vi "niFPGA 3phasePLL.vi"(0 "input (phase value)":T2, 1 "reset":bool, 5 "PI gains":T1={"proportional gain (Kp)"=12.0, "integral gain (Ki)"=200.0}, 7 "anti-windup gain (Ka)":fxp<+,16,9>=200.0, 12 "dt":fxp<+,24,-5>=9.999983012676239e-05) -> (3 "frequency":fxp<+,32,8> format="%.27g", 4 "phase (pi)":fxp<+/-,32,1> format="%.32g", 6 "sin(phase)":fxp<+/-,32,2> format="%.31g", 8 "cos(phase)":fxp<+/-,32,2> format="%.31g")   [LabVIEW 2017]
doc: "Tracks the <B>phase</B> and <B>frequency</B> of a three-phase signal. This operation is useful for FPGA control applications of a three-phase system. The output <B>phase</B> of the 3-Phase Phase-Locked Loop is in pi radians.\n\nTo define the <B>Input mode</B>, double-click this Express VI and use the <B>Input mode</B> control to specify phase value input--<B>input (phase value)</B> or line value input--<B>input (line value)</B>. \n\n\n\nUse this VI in a While Loop."
uses:
  <vilib>/rvi/FXPMathLib/FxpMul/XNode/nifxpmath_Multiplier.xnode
  <vilib>/rvi/FXPMathLib/sim/FxpSim.dll
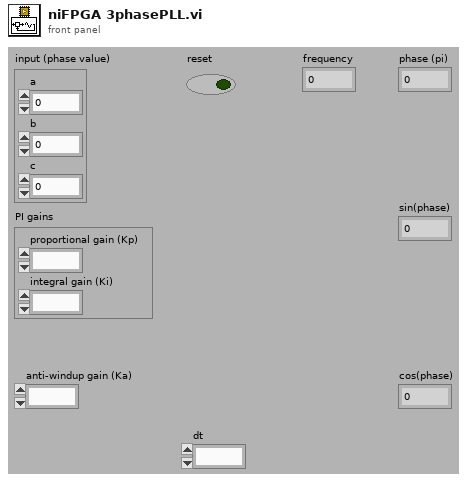
[diagram p1: front panel]
types:
  T1 = cluster{"proportional gain (Kp)":fxp<+,16,6>, "integral gain (Ki)":fxp<+,16,9>}
  T2 = cluster{"a":fxp<+/-,32,8>, "b":fxp<+/-,32,8>, "c":fxp<+/-,32,8>}
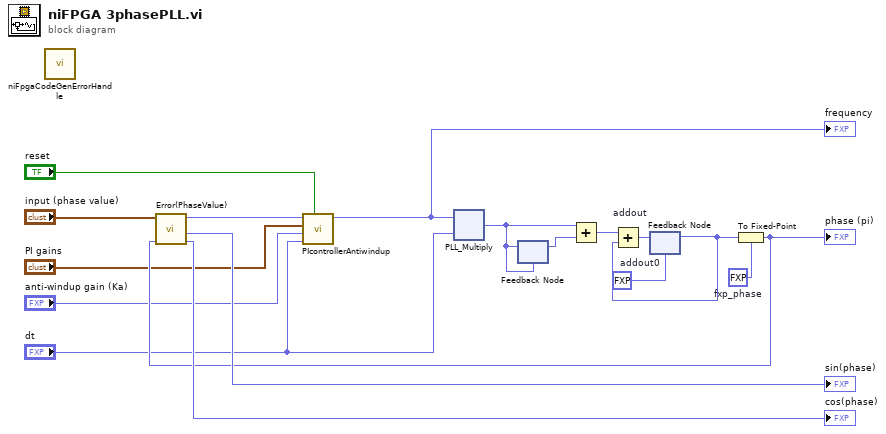
[diagram p0: block diagram]
diagram:
  w14 = fxp<+/-,43,1> 0.0  # addout0
  w16 = fxp<+/-,32,1> 0.0  # fxp_phase
  n1 = call <vilib>:"niFpgaCodeGenErrorHandle.vi"() -> ()  [unwired: 1 in]
  n2 = feedback #1(w14) -> (w17:fxp<+/-,43,1>)
  n3 = To Fixed-Point(fixed-point type=w16, number=w17) -> (fixed-point=w7:fxp<+/-,32,1>)
  "phase (pi)" <- w7
  n4 = call "Error(PhaseValue).vi"("estimated theta"=w7, "phase value"="input (phase value)") -> ("cos(theta)"=→"cos(phase)":fxp<+/-,32,2>, "sin(theta)"=→"sin(phase)":fxp<+/-,32,2>, "error"=w6:fxp<+/-,32,10>)  [unwired: 7 in]
  n5 = call "PIcontrollerAntiwindup.vi"("reset"="reset", "dt"="dt", "anti-windup gain (Ka)"="anti-windup gain (Ka)", "PI gains"="PI gains", "error"=w6) -> ("output"=w2:fxp<+,32,8>)  [unwired: 6 in]
  "frequency" <- w2
  n6 = xnode "PLL_Multiply"("x"=w2, "y"="dt") -> ("x*y"=w13:fxp<+/-,43,1>)
  n7 = feedback #2(w13) -> (w11:fxp<+/-,43,1>)
  n8 = feedback-in #2(w13) -> ()
  n9 = Add(x=w13, y=w11) -> (x+y=w12:fxp<+/-,44,2>)
  n10 = Add "addout"(x=w12, y=w17) -> (x+y=w15:fxp<+/-,43,1>)
  n11 = feedback-in #1(w15) -> ()
